vi "VIve LabVIEW_Simple RGB_U32 to Color[4].vi"(2 "False state  RGB_U32 2":u32(colorbox)=9539985, 3 "True state RGB_U32":u32(colorbox)=13750737) -> (0 "Colors[4]":cluster{u32, u32}[](array[cluster])=[{12966636, 0}])   [LabVIEW 2009]
doc: "This VI sets the True and False state colors.\n\nVIve LabVIEW"
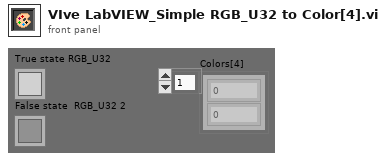
[diagram p1: front panel]
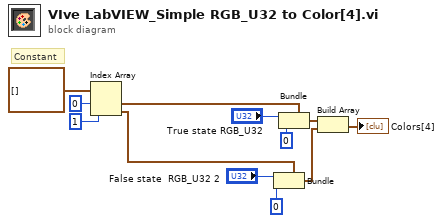
[diagram p0: block diagram]
diagram:
  # "Constant"
  n1 = Index Array(array=cluster{u32, u32}[] [] ("Colors [4]"), index #1=0 ("index"), index #2=1 ("index")) -> (element #1=w12:cluster{u32, u32}, element #2=w4:cluster{u32, u32})
  n2 = Bundle(cluster=w4, "False state  RGB_U32 2", u32 0 ("element")) -> (w2:cluster{u32, u32})
  n3 = Bundle(cluster=w12, "True state RGB_U32", u32 0 ("element")) -> (w3:cluster{u32, u32})
  n4 = Build Array(w3, w2) -> (→"Colors[4]":cluster{u32, u32}[])
